vi "nanocal -- nuclear schottky fit V4.vi"() -> ()   [LabVIEW 2020] (continued)
\"B\"-> 12.000000000000  , \"θ\"-> 30.000000000000  |>   , \r\"IDS0302_210831_RAW_cal__sam_\" ->   <| \"ζ\"->  0.072634365939  , \"τ1\"-> 0.028637109000  , \"τS\"-> 0.065061142288  , \"τN\"-> 0.040304243071  , \"τC\"-> 0.001622979999  , \"κ0\"-> 0.000000001498  , \"mm1\"-> 0.000000000000  , \"mm2\"-> 0.000000000000  , \"mm3\"-> 0.000000000000  , \"T\"->  0.250000000000  , \"B\"-> 12.000000000000  , \"θ\"-> 30.000000000000  |>   , \r\"IDS0303_210831_RAW_cal__ref_\" ->   <| \"ζ\"->  0.210185455037  , \"τ1\"-> 0.035884437188  , \"τS\"-> 0.076269858590  , \"τN\"-> 0.100000000000  , \"τC\"-> 0.001092094788  , \"κ0\"-> 0.000000001049  , \"mm1\"-> 0.000000000000  , \"mm2\"-> 0.000000000000  , \"mm3\"-> 0.000000000000  , \"T\"->  0.200000000000  , \"B\"-> 12.000000000000  , \"θ\"-> 30.000000000000  |>   , \r\"IDS0303_210831_RAW_cal__sam_\" ->   <| \"ζ\"->  0.128615765969  , \"τ1\"-> 0.032665502211  , \"τS\"-> 0.082694869013  , \"τN\"-> 0.105788373632  , \"τC\"-> 0.001439686784  , \"κ0\"-> 0.000000001168  , \"mm1\"-> 0.000000000000  , \"mm2\"-> 0.000000000000  , \"mm3\"-> 0.000000000000  , \"T\"->  0.200000000000  , \"B\"-> 12.000000000000  , \"θ\"-> 30.000000000000  |>   , \r\"IDS0304_210831_RAW_cal__ref_\" ->   <| \"ζ\"->  0.270205686716  , \"τ1\"-> 0.041964859676  , \"τS\"-> 0.093295997771  , \"τN\"-> 0.171907220186  , \"τC\"-> 0.001079705974  , \"κ0\"-> 0.000000000759  , \"mm1\"-> 0.000000000000  , \"mm2\"-> 0.000000000000  , \"mm3\"-> 0.000000000000  , \"T\"->  0.170000000000  , \"B\"-> 12.000000000000  , \"θ\"-> 30.000000000000  |>   , \r\"IDS0304_210831_RAW_cal__sam_\" ->   <| \"ζ\"->  0.156472219566  , \"τ1\"-> 0.031017925061  , \"τS\"-> 0.080872234530  , \"τN\"-> 0.219381306397  , \"τC\"-> 0.001437792153  , \"κ0\"-> 0.000000000867  , \"mm1\"-> 0.000000000000  , \"mm2\"-> 0.000000000000  , \"mm3\"-> 0.000000000000  , \"T\"->  0.170000000000  , \"B\"-> 12.000000000000  , \"θ\"-> 30.000000000000  |>   , \r\"IDS0305_210831_RAW_cal__ref_\" ->   <| \"ζ\"->  0.288872243536  , \"τ1\"-> 0.043051365220  , \"τS\"-> 0.113757726379  , \"τN\"-> 0.232280670982  , \"τC\"-> 0.001075362358  , \"κ0\"-> 0.000000000648  , \"mm1\"-> 0.000000000000  , \"mm2\"-> 0.000000000000  , \"mm3\"-> 0.000000000000  , \"T\"->  0.160000000000  , \"B\"-> 12.000000000000  , \"θ\"-> 30.000000000000  |>   , \r\"IDS0305_210831_RAW_cal__sam_\" ->   <| \"ζ\"->  0.162585495535  , \"τ1\"-> 0.037883389730  , \"τS\"-> 0.086562863191  , \"τN\"-> 0.241872534356  , \"τC\"-> 0.001506143871  , \"κ0\"-> 0.000000000791  , \"mm1\"-> 0.000000000000  , \"mm2\"-> 0.000000000000  , \"mm3\"-> 0.000000000000  , \"T\"->  0.160000000000  , \"B\"-> 12.000000000000  , \"θ\"-> 30.000000000000  |>   , \r\"IDS0306_210831_RAW_cal__ref_\" ->   <| \"ζ\"->  0.013593052641  , \"τ1\"-> 0.010989385662  , \"τS\"-> 0.007947176041  , \"τN\"-> 0.000037757079  , \"τC\"-> 0.003572854733  , \"κ0\"-> 0.000000023548  , \"mm1\"-> 0.000000000000  , \"mm2\"-> 0.000000000000  , \"mm3\"-> 0.000000000000  , \"T\"->  3.100000000000  , \"B\"-> 12.000000000000  , \"θ\"-> 30.000000000000  |>   , \r\"IDS0306_210831_RAW_cal__sam_\" ->   <| \"ζ\"->  0.010111127240  , \"τ1\"-> 0.020788755574  , \"τS\"-> 0.009968978424  , \"τN\"-> 0.000077788811  , \"τC\"-> 0.004598584548  , \"κ0\"-> 0.000000024346  , \"mm1\"-> 0.000000000000  , \"mm2\"-> 0.000000000000  , \"mm3\"-> 0.000000000000  , \"T\"->  3.100000000000  , \"B\"-> 12.000000000000  , \"θ\"-> 30.000000000000  |>   , \r\"IDS0310_210901_RAW_cal__ref_\" ->   <| \"ζ\"->  0.308289315544  , \"τ1\"-> 0.054346075620  , \"τS\"-> 0.066318547481  , \"τN\"-> 0.209207967486  , \"τC\"-> 0.001005266633  , \"κ0\"-> 0.000000000648  , \"mm1\"-> 0.000000000000  , \"mm2\"-> 0.000000000000  , \"mm3\"-> 0.000000000000  , \"T\"->  0.157000000000  , \"B\"-> 12.000000000000  , \"θ\"-> 45.000000000000  |>   , \r\"IDS0310_210901_RAW_cal__sam_\" ->   <| \"ζ\"->  0.295520923520  , \"τ1\"-> 0.054772440405  , \"τS\"-> 0.071814005451  , \"τN\"-> 0.249593767169  , \"τC\"-> 0.001103632155  , \"κ0\"-> 0.000000000625  , \"mm1\"-> 0.000000000000  , \"mm2\"-> 0.000000000000  , \"mm3\"-> 0.000000000000  , \"T\"->  0.157000000000  , \"B\"-> 12.000000000000  , \"θ\"-> 45.000000000000  |>   , \r\"IDS0311_210901_RAW_cal__ref_\" ->   <| \"ζ\"->  0.509291398058  , \"τ1\"-> 0.072489311123  , \"τS\"-> 0.090971238975  , \"τN\"-> 0.493344947632  , \"τC\"-> 0.000983845591  , \"κ0\"-> 0.000000000427  , \"mm1\"-> 0.000000000000  , \"mm2\"-> 0.000000000000  , \"mm3\"-> 0.000000000000  , \"T\"->  0.120000000000  , \"B\"-> 12.000000000000  , \"θ\"-> 45.000000000000  |>   , \r\"IDS0311_210901_RAW_cal__sam_\" ->   <| \"ζ\"->  0.523545279740  , \"τ1\"-> 0.065613539167  , \"τS\"-> 0.100000000000  , \"τN\"-> 0.424083114177  , \"τC\"-> 0.000911255863  , \"κ0\"-> 0.000000000418  , \"mm1\"-> 0.000000000000  , \"mm2\"-> 0.000000000000  , \"mm3\"-> 0.000000000000  , \"T\"->  0.120000000000  , \"B\"-> 12.000000000000  , \"θ\"-> 45.000000000000  |>   , \r\"IDS0312_210901_RAW_cal__ref_\" ->   <| \"ζ\"->  0.255987747016  , \"τ1\"-> 0.050915418179  , \"τS\"-> 0.056322890077  , \"τN\"-> 0.162539494258  , \"τC\"-> 0.001014478551  , \"κ0\"-> 0.000000000752  , \"mm1\"-> 0.000000000000  , \"mm2\"-> 0.000000000000  , \"mm3\"-> 0.000000000000  , \"T\"->  0.170000000000  , \"B\"-> 12.000000000000  , \"θ\"-> 45.000000000000  |>   , \r\"IDS0312_210901_RAW_cal__sam_\" ->   <| \"ζ\"->  0.273742116471  , \"τ1\"-> 0.052262909995  , \"τS\"-> 0.060554036646  , \"τN\"-> 0.154269705680  , \"τC\"-> 0.001074144337  , \"κ0\"-> 0.000000000753  , \"mm1\"-> 0.000000000000  , \"mm2\"-> 0.000000000000  , \"mm3\"-> 0.000000000000  , \"T\"->  0.170000000000  , \"B\"-> 12.000000000000  , \"θ\"-> 45.000000000000  |>   , \r\"IDS0313_210901_RAW_cal__ref_\" ->   <| \"ζ\"->  0.214174227031  , \"τ1\"-> 0.045371966885  , \"τS\"-> 0.046160741010  , \"τN\"-> 0.090352099204  , \"τC\"-> 0.001077653985  , \"κ0\"-> 0.000000001047  , \"mm1\"-> 0.000000000000  , \"mm2\"-> 0.000000000000  , \"mm3\"-> 0.000000000000  , \"T\"->  0.200000000000  , \"B\"-> 12.000000000000  , \"θ\"-> 45.000000000000  |>   , \r\"IDS0313_210901_RAW_cal__sam_\" ->   <| \"ζ\"->  0.215688135788  , \"τ1\"-> 0.043710888546  , \"τS\"-> 0.044756474141  , \"τN\"-> 0.090222547904  , \"τC\"-> 0.001049781785  , \"κ0\"-> 0.000000001047  , \"mm1\"-> 0.000000000000  , \"mm2\"-> 0.000000000000  , \"mm3\"-> 0.000000000000  , \"T\"->  0.200000000000  , \"B\"-> 12.000000000000  , \"θ\"-> 45.000000000000  |>   , \r\"IDS0314_210901_RAW_cal__ref_\" ->   <| \"ζ\"->  0.121938807235  , \"τ1\"-> 0.034207371807  , \"τS\"-> 0.036720955072  , \"τN\"-> 0.033836278502  , \"τC\"-> 0.001295467245  , \"κ0\"-> 0.000000001354  , \"mm1\"-> 0.000000000000  , \"mm2\"-> 0.000000000000  , \"mm3\"-> 0.000000000000  , \"T\"->  0.255000000000  , \"B\"-> 12.000000000000  , \"θ\"-> 45.000000000000  |>   , \r\"IDS0314_210901_RAW_cal__sam_\" ->   <| \"ζ\"->  0.118583992968  , \"τ1\"-> 0.035232851003  , \"τS\"-> 0.037458022816  , \"τN\"-> 0.033724509363  , \"τC\"-> 0.001440922263  , \"κ0\"-> 0.000000001360  , \"mm1\"-> 0.000000000000  , \"mm2\"-> 0.000000000000  , \"mm3\"-> 0.000000000000  , \"T\"->  0.255000000000  , \"B\"-> 12.000000000000  , \"θ\"-> 45.000000000000  |>   , \r\"IDS0315_210901_RAW_cal__ref_\" ->   <| \"ζ\"->  0.083994348522  , \"τ1\"-> 0.028454655874  , \"τS\"-> 0.032547522861  , \"τN\"-> 0.016695645368  , \"τC\"-> 0.001519868181  , \"κ0\"-> 0.000000001732  , \"mm1\"-> 0.000000000000  , \"mm2\"-> 0.000000000000  , \"mm3\"-> 0.000000000000  , \"T\"->  0.300000000000  , \"B\"-> 12.000000000000  , \"θ\"-> 45.000000000000  |>   , \r\"IDS0315_210901_RAW_cal__sam_\" ->   <| \"ζ\"->  0.085152769414  , \"τ1\"-> 0.029001116263  , \"τS\"-> 0.032604663993  , \"τN\"-> 0.016878763935  , \"τC\"-> 0.001443524845  , \"κ0\"-> 0.000000001728  , \"mm1\"-> 0.000000000000  , \"mm2\"-> 0.000000000000  , \"mm3\"-> 0.000000000000  , \"T\"->  0.300000000000  , \"B\"-> 12.000000000000  , \"θ\"-> 45.000000000000  |>   , \r\"IDS0316_210901_RAW_cal__ref_\" ->   <| \"ζ\"->  0.061161812807  , \"τ1\"-> 0.025679940958  , \"τS\"-> 0.030186846656  , \"τN\"-> 0.009745770789  , \"τC\"-> 0.001942458613  , \"κ0\"-> 0.000000002119  , \"mm1\"-> 0.000000000000  , \"mm2\"-> 0.000000000000  , \"mm3\"-> 0.000000000000  , \"T\"->  0.360000000000  , \"B\"-> 12.000000000000  , \"θ\"-> 45.000000000000  |>   , \r\"IDS0316_210901_RAW_cal__sam_\" ->   <| \"ζ\"->  0.061011838044  , \"τ1\"-> 0.025440548989  , \"τS\"-> 0.030028053978  , \"τN\"-> 0.010140731955  , \"τC\"-> 0.001895079687  , \"κ0\"-> 0.000000002115  , \"mm1\"-> 0.000000000000  , \"mm2\"-> 0.000000000000  , \"mm3\"-> 0.000000000000  , \"T\"->  0.360000000000  , \"B\"-> 12.000000000000  , \"θ\"-> 45.000000000000  |>   , \r\"IDS0317_210901_RAW_cal__ref_\" ->   <| \"ζ\"->  0.047188818117  , \"τ1\"-> 0.023281630947  , \"τS\"-> 0.027595934693  , \"τN\"-> 0.005357909158  , \"τC\"-> 0.002405018291  , \"κ0\"-> 0.000000002634  , \"mm1\"-> 0.000000000000  , \"mm2\"-> 0.000000000000  , \"mm3\"-> 0.000000000000  , \"T\"->  0.430000000000  , \"B\"-> 12.000000000000  , \"θ\"-> 45.000000000000  |>   , \r\"IDS0317_210901_RAW_cal__sam_\" ->   <| \"ζ\"->  0.046686299518  , \"τ1\"-> 0.021011215626  , \"τS\"-> 0.027633142317  , \"τN\"-> 0.005348477555  , \"τC\"-> 0.002098477650  , \"κ0\"-> 0.000000002635  , \"mm1\"-> 0.000000000000  , \"mm2\"-> 0.000000000000  , \"mm3\"-> 0.000000000000  , \"T\"->  0.430000000000  , \"B\"-> 12.000000000000  , \"θ\"-> 45.000000000000  |>   , \r\"IDS0318_210901_RAW_cal__ref_\" ->   <| \"ζ\"->  0.037288247068  , \"τ1\"-> 0.020701608824  , \"τS\"-> 0.025512873362  , \"τN\"-> 0.002622201076  , \"τC\"-> 0.002753838304  , \"κ0\"-> 0.000000003290  , \"mm1\"-> 0.000000000000  , \"mm2\"-> 0.000000000000  , \"mm3\"-> 0.000000000000  , \"T\"->  0.530000000000  , \"B\"-> 12.000000000000  , \"θ\"-> 45.000000000000  |>   , \r\"IDS0318_210901_RAW_cal__sam_\" ->   <| \"ζ\"->  0.035204330012  , \"τ1\"-> 0.021011523093  , \"τS\"-> 0.025247316079  , \"τN\"-> 0.002718647875  , \"τC\"-> 0.003091727575  , \"κ0\"-> 0.000000003296  , \"mm1\"-> 0.000000000000  , \"mm2\"-> 0.000000000000  , \"mm3\"-> 0.000000000000  , \"T\"->  0.530000000000  , \"B\"-> 12.000000000000  , \"θ\"-> 45.000000000000  |>   , \r\"IDS0319_210901_RAW_cal__ref_\" ->   <| \"ζ\"->  0.029057248634  , \"τ1\"-> 0.018506971535  , \"τS\"-> 0.023958337181  , \"τN\"-> 0.001609750825  , \"τC\"-> 0.003041346082  , \"κ0\"-> 0.000000003909  , \"mm1\"-> 0.000000000000  , \"mm2\"-> 0.000000000000  , \"mm3\"-> 0.000000000000  , \"T\"->  0.620000000000  , \"B\"-> 12.000000000000  , \"θ\"-> 45.000000000000  |>   , \r\"IDS0319_210901_RAW_cal__sam_\" ->   <| \"ζ\"->  0.030862035723  , \"τ1\"-> 0.019328530751  , \"τS\"-> 0.023568572597  , \"τN\"-> 0.001701966614  , \"τC\"-> 0.003453790534  , \"κ0\"-> 0.000000003906  , \"mm1\"-> 0.000000000000  , \"mm2\"-> 0.000000000000  , \"mm3\"-> 0.000000000000  , \"T\"->  0.620000000000  , \"B\"-> 12.000000000000  , \"θ\"-> 45.000000000000  |>   , \r\"IDS0320_210901_RAW_cal__ref_\" ->   <| \"ζ\"->  0.022379315068  , \"τ1\"-> 0.015662672554  , \"τS\"-> 0.020062485201  , \"τN\"-> 0.000750608517  , \"τC\"-> 0.004162319228  , \"κ0\"-> 0.000000005449  , \"mm1\"-> 0.000000000000  , \"mm2\"-> 0.000000000000  , \"mm3\"-> 0.000000000000  , \"T\"->  0.830000000000  , \"B\"-> 12.000000000000  , \"θ\"-> 45.000000000000  |>   , \r\"IDS0320_210901_RAW_cal__sam_\" ->   <| \"ζ\"->  0.023591124045  , \"τ1\"-> 0.014910006225  , \"τS\"-> 0.019342950404  , \"τN\"-> 0.000752972387  , \"τC\"-> 0.004900413232  , \"κ0\"-> 0.000000005453  , \"mm1\"-> 0.000000000000  , \"mm2\"-> 0.000000000000  , \"mm3\"-> 0.000000000000  , \"T\"->  0.830000000000  , \"B\"-> 12.000000000000  , \"θ\"-> 45.000000000000  |>   , \r\"IDS0321_210901_RAW_cal__ref_\" ->   <| \"ζ\"->  0.020614746765  , \"τ1\"-> 0.013682065369  , \"τS\"-> 0.016105139108  , \"τN\"-> 0.000397734649  , \"τC\"-> 0.005005824303  , \"κ0\"-> 0.000000007592  , \"mm1\"-> 0.000000000000  , \"mm2\"-> 0.000000000000  , \"mm3\"-> 0.000000000000  , \"T\"->  1.130000000000  , \"B\"-> 12.000000000000  , \"θ\"-> 45.000000000000  |>   , \r\"IDS0321_210901_RAW_cal__sam_\" ->   <| \"ζ\"->  0.020215154826  , \"τ1\"-> 0.014105227254  , \"τS\"-> 0.015660924043  , \"τN\"-> 0.000525137036  , \"τC\"-> 0.005447728357  , \"κ0\"-> 0.000000007594  , \"mm1\"-> 0.000000000000  , \"mm2\"-> 0.000000000000  , \"mm3\"-> 0.000000000000  , \"T\"->  1.130000000000  , \"B\"-> 12.000000000000  , \"θ\"-> 45.000000000000  |>   , \r\"IDS0322_210901_RAW_cal__ref_\" ->   <| \"ζ\"->  0.019557893298  , \"τ1\"-> 0.012446212333  , \"τS\"-> 0.011139553358  , \"τN\"-> 0.000114229396  , \"τC\"-> 0.005115315079  , \"κ0\"-> 0.000000013115  , \"mm1\"-> 0.000000000000  , \"mm2\"-> 0.000000000000  , \"mm3\"-> 0.000000000000  , \"T\"->  1.900000000000  , \"B\"-> 12.000000000000  , \"θ\"-> 45.000000000000  |>   , \r\"IDS0322_210901_RAW_cal__sam_\" ->   <| \"ζ\"->  0.018090572724  , \"τ1\"-> 0.013314780956  , \"τS\"-> 0.010820835010  , \"τN\"-> 0.000265552167  , \"τC\"-> 0.005393540417  , \"κ0\"-> 0.000000013100  , \"mm1\"-> 0.000000000000  , \"mm2\"-> 0.000000000000  , \"mm3\"-> 0.000000000000  , \"T\"->  1.900000000000  , \"B\"-> 12.000000000000  , \"θ\"-> 45.000000000000  |>   , \r\"IDS0323_210901_RAW_cal__ref_\" ->   <| \"ζ\"->  0.018290634783  , \"τ1\"-> 0.011707989393  , \"τS\"-> 0.007391181448  , \"τN\"-> 0.000042685582  , \"τC\"-> 0.004638632451  , \"κ0\"-> 0.000000023525  , \"mm1\"-> 0.000000000000  , \"mm2\"-> 0.000000000000  , \"mm3\"-> 0.000000000000  , \"T\"->  3.100000000000  , \"B\"-> 12.000000000000  , \"θ\"-> 45.000000000000  |>   , \r\"IDS0323_210901_RAW_cal__sam_\" ->   <| \"ζ\"->  0.019438138135  , \"τ1\"-> 0.013521019406  , \"τS\"-> 0.007253169401  , \"τN\"-> 0.000154824830  , \"τC\"-> 0.004746579385  , \"κ0\"-> 0.000000023466  , \"mm1\"-> 0.000000000000  , \"mm2\"-> 0.000000000000  , \"mm3\"-> 0.000000000000  , \"T\"->  3.100000000000  , \"B\"-> 12.000000000000  , \"θ\"-> 45.000000000000  |>   , \r\"IDS0324_210901_RAW_cal__ref_\" ->   <| \"ζ\"->  0.016342153608  , \"τ1\"-> 0.012470308436  , \"τS\"-> 0.004793459347  , \"τN\"-> 0.000012881713  , \"τC\"-> 0.003213848745  , \"κ0\"-> 0.000000058321  , \"mm1\"-> 0.000000000000  , \"mm2\"-> 0.000000000000  , \"mm3\"-> 0.000000000000  , \"T\"->  5.700000000000  , \"B\"-> 12.000000000000  , \"θ\"-> 45.000000000000  |>   , \r\"IDS0324_210901_RAW_cal__sam_\" ->   <| \"ζ\"->  0.018573189054  , \"τ1\"-> 0.013304612245  , \"τS\"-> 0.003723860844  , \"τN\"-> 0.000084829442  , \"τC\"-> 0.004309703632  , \"κ0\"-> 0.000000058362  , \"mm1\"-> 0.000000000000  , \"mm2\"-> 0.000000000000  , \"mm3\"-> 0.000000000000  , \"T\"->  5.700000000000  , \"B\"-> 12.000000000000  , \"θ\"-> 45.000000000000  |>   , \r\"IDS0330_210901_RAW_cal__ref_\" ->   <| \"ζ\"->  0.000000000000  , \"τ1\"-> 0.000000000000  , \"τS\"-> 0.000000000000  , \"τN\"-> 0.000000000000  , \"τC\"-> 0.000000000000  , \"κ0\"-> 0.000000000000  , \"mm1\"-> 0.000000000000  , \"mm2\"-> 0.000000000000  , \"mm3\"-> 0.000000000000  , \"T\"->  0.197000000000  , \"B\"-> 1.000000000000  , \"θ\"-> 90.000000000000  |>   , \r\"IDS0330_210901_RAW_cal__sam_\" ->   <| \"ζ\"->  0.000000000000  , \"τ1\"-> 0.000000000000  , \"τS\"-> 0.000000000000  , \"τN\"-> 0.000000000000  , \"τC\"-> 0.000000000000  , \"κ0\"-> 0.000000000000  , \"mm1\"-> 0.000000000000  , \"mm2\"-> 0.000000000000  , \"mm3\"-> 0.000000000000  , \"T\"->  0.197000000000  , \"B\"-> 1.000000000000  , \"θ\"-> 90.000000000000  |>   , \r\"IDS0331_210901_RAW_cal__ref_\" ->   <| \"ζ\"->  0.000000000000  , \"τ1\"-> 0.000000000000  , \"τS\"-> 0.000000000000  , \"τN\"-> 0.000000000000  , \"τC\"-> 0.000000000000  , \"κ0\"-> 0.000000000000  , \"mm1\"-> 0.000000000000  , \"mm2\"-> 0.000000000000  , \"mm3\"-> 0.000000000000  , \"T\"->  0.197000000000  , \"B\"-> 2.000000000000  , \"θ\"-> 90.000000000000  |>   , \r\"IDS0331_210901_RAW_cal__sam_\" ->   <| \"ζ\"->  0.000000000000  , \"τ1\"-> 0.000000000000  , \"τS\"-> 0.000000000000  , \"τN\"-> 0.000000000000  , \"τC\"-> 0.000000000000  , \"κ0\"-> 0.000000000000  , \"mm1\"-> 0.000000000000  , \"mm2\"-> 0.000000000000  , \"mm3\"-> 0.000000000000  , \"T\"->  0.197000000000  , \"B\"-> 2.000000000000  , \"θ\"-> 90.000000000000  |>   , \r\"IDS0335_210904_RAW_cal__ref_\" ->   <| \"ζ\"->  0.205498470214  , \"τ1\"-> 0.028285232133  , \"τS\"-> 0.084091632013  , \"τN\"-> 0.011152237921  , \"τC\"-> 0.001130624685  , \"κ0\"-> 0.000000001029  , \"mm1\"-> 0.000000000000  , \"mm2\"-> 0.000000000000  , \"mm3\"-> 0.000000000000  , \"T\"->  0.197000000000  , \"B\"-> 5.000000000000  , \"θ\"-> 90.000000000000  |>   , \r\"IDS0335_210904_RAW_cal__sam_\" ->   <| \"ζ\"->  0.126020527573  , \"τ1\"-> 0.019611338518  , \"τS\"-> 0.107746773503  , \"τN\"-> 0.016174642295  , \"τC\"-> 0.001503883282  , \"κ0\"-> 0.000000001131  , \"mm1\"-> 0.000000000000  , \"mm2\"-> 0.000000000000  , \"mm3\"-> 0.000000000000  , \"T\"->  0.197000000000  , \"B\"-> 5.000000000000  , \"θ\"-> 90.000000000000  |>   , \r\"IDS0336_210904_RAW_cal__ref_\" ->   <| \"ζ\"->  0.375717568518  , \"τ1\"-> 0.027671879302  , \"τS\"-> 0.199029510980  , \"τN\"-> 0.083427621052  , \"τC\"-> 0.001244823236  , \"κ0\"-> 0.000000000403  , \"mm1\"-> 0.000000000000  , \"mm2\"-> 0.000000000000  , \"mm3\"-> 0.000000000000  , \"T\"->  0.122000000000  , \"B\"-> 5.000000000000  , \"θ\"-> 90.000000000000  |>   , \r\"IDS0336_210904_RAW_cal__sam_\" ->   <| \"ζ\"->  0.199029510980  , \"τ1\"-> 0.022641147583  , \"τS\"-> 0.278068103221  , \"τN\"-> 0.092231648139  , \"τC\"-> 0.001612694918  , \"κ0\"-> 0.000000000500  , \"mm1\"-> 0.000000000000  , \"mm2\"-> 0.000000000000  , \"mm3\"-> 0.000000000000  , \"T\"->  0.122000000000  , \"B\"-> 5.000000000000  , \"θ\"-> 90.000000000000  |>   , \r\"IDS0337_210904_RAW_cal__ref_\" ->   <| \"ζ\"->  0.292356831523  , \"τ1\"-> 0.026984636460  , \"τS\"-> 0.124002379909  , \"τN\"-> 0.023667494338  , \"τC\"-> 0.001131071001  , \"κ0\"-> 0.000000000646  , \"mm1\"-> 0.000000000000  , \"mm2\"-> 0.000000000000  , \"mm3\"-> 0.000000000000  , \"T\"->  0.157000000000  , \"B\"-> 5.000000000000  , \"θ\"-> 90.000000000000  |>   , \r\"IDS0337_210904_RAW_cal__sam_\" ->   <| \"ζ\"->  0.176509782472  , \"τ1\"-> 0.020702853275  , \"τS\"-> 0.157609352978  , \"τN\"-> 0.029245874633  , \"τC\"-> 0.001454463496  , \"κ0\"-> 0.000000000745  , \"mm1\"-> 0.000000000000  , \"mm2\"-> 0.000000000000  , \"mm3\"-> 0.000000000000  , \"T\"->  0.157000000000  , \"B\"-> 5.000000000000  , \"θ\"-> 90.000000000000  |>   , \r\"IDS0338_210904_RAW_cal__ref_\" ->   <| \"ζ\"->  0.269210160049  , \"τ1\"-> 0.027533256233  , \"τS\"-> 0.109874895668  , \"τN\"-> 0.015552411517  , \"τC\"-> 0.001074349295  , \"κ0\"-> 0.000000000732  , \"mm1\"-> 0.000000000000  , \"mm2\"-> 0.000000000000  , \"mm3\"-> 0.000000000000  , \"T\"->  0.170000000000  , \"B\"-> 5.000000000000  , \"θ\"-> 90.000000000000  |>   , \r\"IDS0338_210904_RAW_cal__sam_\" ->   <| \"ζ\"->  0.165922290438  , \"τ1\"-> 0.020050534769  , \"τS\"-> 0.138657975356  , \"τN\"-> 0.024093470374  , \"τC\"-> 0.001416071995  , \"κ0\"-> 0.000000000842  , \"mm1\"-> 0.000000000000  , \"mm2\"-> 0.000000000000  , \"mm3\"-> 0.000000000000  , \"T\"->  0.170000000000  , \"B\"-> 5.000000000000  , \"θ\"-> 90.000000000000  |>   , \r\"IDS0339_210904_RAW_cal__ref_\" ->   <| \"ζ\"->  0.119201785186  , \"τ1\"-> 0.025848962424  , \"τS\"-> 0.059947037778  , \"τN\"-> 0.005199563600  , \"τC\"-> 0.001300898921  , \"κ0\"-> 0.000000001342  , \"mm1\"-> 0.000000000000  , \"mm2\"-> 0.000000000000  , \"mm3\"-> 0.000000000000  , \"T\"->  0.255000000000  , \"B\"-> 5.000000000000  , \"θ\"-> 90.000000000000  |>   , \r\"IDS0339_210904_RAW_cal__sam_\" ->   <| \"ζ\"->  0.071445093965  , \"τ1\"-> 0.018200134719  , \"τS\"-> 0.077244369618  , \"τN\"-> 0.007618519700  , \"τC\"-> 0.001758409609  , \"κ0\"-> 0.000000001475  , \"mm1\"-> 0.000000000000  , \"mm2\"-> 0.000000000000  , \"mm3\"-> 0.000000000000  , \"T\"->  0.255000000000  , \"B\"-> 5.000000000000  , \"θ\"-> 90.000000000000  |>   , \r\"IDS0340_210904_RAW_cal__ref_\" ->   <| \"ζ\"->  0.082683893253  , \"τ1\"-> 0.024702194699  , \"τS\"-> 0.049753720072  , \"τN\"-> 0.002517387539  , \"τC\"-> 0.001542602546  , \"κ0\"-> 0.000000001719  , \"mm1\"-> 0.000000000000  , \"mm2\"-> 0.000000000000  , \"mm3\"-> 0.000000000000  , \"T\"->  0.308000000000  , \"B\"-> 5.000000000000  , \"θ\"-> 90.000000000000  |>   , \r\"IDS0340_210904_RAW_cal__sam_\" ->   <| \"ζ\"->  0.049152938826  , \"τ1\"-> 0.019216107215  , \"τS\"-> 0.064101941953  , \"τN\"-> 0.003869712687  , \"τC\"-> 0.002203680801  , \"κ0\"-> 0.000000001878  , \"mm1\"-> 0.000000000000  , \"mm2\"-> 0.000000000000  , \"mm3\"-> 0.000000000000  , \"T\"->  0.308000000000  , \"B\"-> 5.000000000000  , \"θ\"-> 90.000000000000  |>   , \r\"IDS0341_210904_RAW_cal__ref_\" ->   <| \"ζ\"->  0.059616809183  , \"τ1\"-> 0.023939570797  , \"τS\"-> 0.042653632086  , \"τN\"-> 0.001786288241  , \"τC\"-> 0.001975926031  , \"κ0\"-> 0.000000002092  , \"mm1\"-> 0.000000000000  , \"mm2\"-> 0.000000000000  , \"mm3\"-> 0.000000000000  , \"T\"->  0.360000000000  , \"B\"-> 5.000000000000  , \"θ\"-> 90.000000000000  |>   , \r\"IDS0341_210904_RAW_cal__sam_\" ->   <| \"ζ\"->  0.036041476168  , \"τ1\"-> 0.019203470752  , \"τS\"-> 0.054931014880  , \"τN\"-> 0.002271152158  , \"τC\"-> 0.002720100083  , \"κ0\"-> 0.000000002280  , \"mm1\"-> 0.000000000000  , \"mm2\"-> 0.000000000000  , \"mm3\"-> 0.000000000000  , \"T\"->  0.360000000000  , \"B\"-> 5.000000000000  , \"θ\"-> 90.000000000000  |>   , \r\"IDS0342_210904_RAW_cal__ref_\" ->   <| \"ζ\"->  0.044217232361  , \"τ1\"-> 0.023574215500  , \"τS\"-> 0.035981580515  , \"τN\"-> 0.001074333911  , \"τC\"-> 0.002351862552  , \"κ0\"-> 0.000000002629  , \"mm1\"-> 0.000000000000  , \"mm2\"-> 0.000000000000  , \"mm3\"-> 0.000000000000  , \"T\"->  0.438000000000  , \"B\"-> 5.000000000000  , \"θ\"-> 90.000000000000  |>   , \r\"IDS0342_210904_RAW_cal__sam_\" ->   <| \"ζ\"->  0.027360242550  , \"τ1\"-> 0.019369895135  , \"τS\"-> 0.046063450687  , \"τN\"-> 0.001549427641  , \"τC\"-> 0.003313507267  , \"κ0\"-> 0.000000002850  , \"mm1\"-> 0.000000000000  , \"mm2\"-> 0.000000000000  , \"mm3\"-> 0.000000000000  , \"T\"->  0.438000000000  , \"B\"-> 5.000000000000  , \"θ\"-> 90.000000000000  |>   , \r\"IDS0343_210904_RAW_cal__ref_\" ->   <| \"ζ\"->  0.035616644679  , \"τ1\"-> 0.021293989016  , \"τS\"-> 0.030504656314  , \"τN\"-> 0.000733387796  , \"τC\"-> 0.002756004742  , \"κ0\"-> 0.000000003268  , \"mm1\"-> 0.000000000000  , \"mm2\"-> 0.000000000000  , \"mm3\"-> 0.000000000000  , \"T\"->  0.530000000000  , \"B\"-> 5.000000000000  , \"θ\"-> 90.000000000000  |>   , \r\"IDS0343_210904_RAW_cal__sam_\" ->   <| \"ζ\"->  0.022691746072  , \"τ1\"-> 0.019361166937  , \"τS\"-> 0.038571137960  , \"τN\"-> 0.001037489181  , \"τC\"-> 0.004002961022  , \"κ0\"-> 0.000000003536  , \"mm1\"-> 0.000000000000  , \"mm2\"-> 0.000000000000  , \"mm3\"-> 0.000000000000  , \"T\"->  0.530000000000  , \"B\"-> 5.000000000000  , \"θ\"-> 90.000000000000  |>   , \r\"IDS0344_210904_RAW_cal__ref_\" ->   <| \"ζ\"->  0.029414072191  , \"τ1\"-> 0.022729389588  , \"τS\"-> 0.026807996891  , \"τN\"-> 0.000501873075  , \"τC\"-> 0.003020821681  , \"κ0\"-> 0.000000003880  , \"mm1\"-> 0.000000000000  , \"mm2\"-> 0.000000000000  , \"mm3\"-> 0.000000000000  , \"T\"->  0.620000000000  , \"B\"-> 5.000000000000  , \"θ\"-> 90.000000000000  |>   , \r\"IDS0344_210904_RAW_cal__sam_\" ->   <| \"ζ\"->  0.018598309928  , \"τ1\"-> 0.019376212159  , \"τS\"-> 0.033569863125  , \"τN\"-> 0.000771760425  , \"τC\"-> 0.004371934540  , \"κ0\"-> 0.000000004218  , \"mm1\"-> 0.000000000000  , \"mm2\"-> 0.000000000000  , \"mm3\"-> 0.000000000000  , \"T\"->  0.620000000000  , \"B\"-> 5.000000000000  , \"θ\"-> 90.000000000000  |>   , \r\"IDS0346_210904_RAW_cal__ref_\" ->   <| \"ζ\"->  0.351410523880  , \"τ1\"-> 0.038660935015  , \"τS\"-> 0.057750106762  , \"τN\"-> 0.192483765517  , \"τC\"-> 0.000883347451  , \"κ0\"-> 0.000000000403  , \"mm1\"-> 0.000000000000  , \"mm2\"-> 0.000000000000  , \"mm3\"-> 0.000000000000  , \"T\"->  0.122000000000  , \"B\"-> 8.000000000000  , \"θ\"-> 90.000000000000  |>   , \r\"IDS0346_210904_RAW_cal__sam_\" ->   <| \"ζ\"->  0.000000000000  , \"τ1\"-> 0.000000000000  , \"τS\"-> 0.000000000000  , \"τN\"-> 0.000000000000  , \"τC\"-> 0.000000000000  , \"κ0\"-> 0.000000000000  , \"mm1\"-> 0.000000000000  , \"mm2\"-> 0.000000000000  , \"mm3\"-> 0.000000000000  , \"T\"->  0.122000000000  , \"B\"-> 8.000000000000  , \"θ\"-> 90.000000000000  |>   , \r\"IDS0347_210906_RAW_cal__ref_\" ->   <| \"ζ\"->  0.282365663511  , \"τ1\"-> 0.039144945999  , \"τS\"-> 0.059953399264  , \"τN\"-> 0.108048405778  , \"τC\"-> 0.001096068963  , \"κ0\"-> 0.000000000641  , \"mm1\"-> 0.000000000000  , \"mm2\"-> 0.000000000000  , \"mm3\"-> 0.000000000000  , \"T\"->  0.157000000000  , \"B\"-> 8.000000000000  , \"θ\"-> 90.000000000000  |>   , \r\"IDS0347_210906_RAW_cal__sam_\" ->   <| \"ζ\"->  0.000000000000  , \"τ1\"-> 0.000000000000  , \"τS\"-> 0.000000000000  , \"τN\"-> 0.000000000000  , \"τC\"-> 0.000000000000  , \"κ0\"-> 0.000000000000  , \"mm1\"-> 0.000000000000  , \"mm2\"-> 0.000000000000  , \"mm3\"-> 0.000000000000  , \"T\"->  0.157000000000  , \"B\"-> 8.000000000000  , \"θ\"-> 90.000000000000  |>   , \r\"IDS0348_210906_RAW_cal__ref_\" ->   <| \"ζ\"->  0.231232733983  , \"τ1\"-> 0.036430431380  , \"τS\"-> 0.054781597050  , \"τN\"-> 0.064844477869  , \"τC\"-> 0.001068830966  , \"κ0\"-> 0.000000000760  , \"mm1\"-> 0.000000000000  , \"mm2\"-> 0.000000000000  , \"mm3\"-> 0.000000000000  , \"T\"->  0.178000000000  , \"B\"-> 8.000000000000  , \"θ\"-> 90.000000000000  |>   , \r\"IDS0348_210906_RAW_cal__sam_\" ->   <| \"ζ\"->  0.000000000000  , \"τ1\"-> 0.000000000000  , \"τS\"-> 0.000000000000  , \"τN\"-> 0.000000000000  , \"τC\"-> 0.000000000000  , \"κ0\"-> 0.000000000000  , \"mm1\"-> 0.000000000000  , \"mm2\"-> 0.000000000000  , \"mm3\"-> 0.000000000000  , \"T\"->  0.178000000000  , \"B\"-> 8.000000000000  , \"θ\"-> 90.000000000000  |>   , \r\"IDS0349_210906_RAW_cal__ref_\" ->   <| \"ζ\"->  0.190485473901  , \"τ1\"-> 0.032323616024  , \"τS\"-> 0.052823523941  , \"τN\"-> 0.036537332757  , \"τC\"-> 0.001181014846  , \"κ0\"-> 0.000000001037  , \"mm1\"-> 0.000000000000  , \"mm2\"-> 0.000000000000  , \"mm3\"-> 0.000000000000  , \"T\"->  0.200000000000  , \"B\"-> 8.000000000000  , \"θ\"-> 90.000000000000  |>   , \r\"IDS0349_210906_RAW_cal__sam_\" ->   <| \"ζ\"->  0.000000000000  , \"τ1\"-> 0.000000000000  , \"τS\"-> 0.000000000000  , \"τN\"-> 0.000000000000  , \"τC\"-> 0.000000000000  , \"κ0\"-> 0.000000000000  , \"mm1\"-> 0.000000000000  , \"mm2\"-> 0.000000000000  , \"mm3\"-> 0.000000000000  , \"T\"->  0.200000000000  , \"B\"-> 8.000000000000  , \"θ\"-> 90.000000000000  |>   , \r\"IDS0350_210906_RAW_cal__ref_\" ->   <| \"ζ\"->  0.118733755426  , \"τ1\"-> 0.027090622935  , \"τS\"-> 0.042154952610  , \"τN\"-> 0.016299612233  , \"τC\"-> 0.001268322773  , \"κ0\"-> 0.000000001347  , \"mm1\"-> 0.000000000000  , \"mm2\"-> 0.000000000000  , \"mm3\"-> 0.000000000000  , \"T\"->  0.260000000000  , \"B\"-> 8.000000000000  , \"θ\"-> 90.000000000000  |>   , \r\"IDS0350_210906_RAW_cal__sam_\" ->   <| \"ζ\"->  0.000000000000  , \"τ1\"-> 0.000000000000  , \"τS\"-> 0.000000000000  , \"τN\"-> 0.000000000000  , \"τC\"-> 0.000000000000  , \"κ0\"-> 0.000000000000  , \"mm1\"-> 0.000000000000  , \"mm2\"-> 0.000000000000  , \"mm3\"-> 0.000000000000  , \"T\"->  0.260000000000  , \"B\"-> 8.000000000000  , \"θ\"-> 90.000000000000  |>   , \r\"IDS0351_210906_RAW_cal__ref_\" ->   <| \"ζ\"->  0.081031099964  , \"τ1\"-> 0.021876847581  , \"τS\"-> 0.037173038366  , \"τN\"-> 0.007845971856  , \"τC\"-> 0.001561862252  , \"κ0\"-> 0.000000001761  , \"mm1\"-> 0.000000000000  , \"mm2\"-> 0.000000000000  , \"mm3\"-> 0.000000000000  , \"T\"->  0.310000000000  , \"B\"-> 8.000000000000  , \"θ\"-> 90.000000000000  |>   , \r\"IDS0351_210906_RAW_cal__sam_\" ->   <| \"ζ\"->  0.000000000000  , \"τ1\"-> 0.000000000000  , \"τS\"-> 0.000000000000  , \"τN\"-> 0.000000000000  , \"τC\"-> 0.000000000000  , \"κ0\"-> 0.000000000000  , \"mm1\"-> 0.000000000000  , \"mm2\"-> 0.000000000000  , \"mm3\"-> 0.000000000000  , \"T\"->  0.310000000000  , \"B\"-> 8.000000000000  , \"θ\"-> 90.000000000000  |>   , \r\"IDS0352_210906_RAW_cal__ref_\" ->   <| \"ζ\"->  0.060336863550  , \"τ1\"-> 0.020607625563  , \"τS\"-> 0.034334079822  , \"τN\"-> 0.004923011954  , \"τC\"-> 0.001895452704  , \"κ0\"-> 0.000000002106  , \"mm1\"-> 0.000000000000  , \"mm2\"-> 0.000000000000  , \"mm3\"-> 0.000000000000  , \"T\"->  0.360000000000  , \"B\"-> 8.000000000000  , \"θ\"-> 90.000000000000  |>   , \r\"IDS0352_210906_RAW_cal__sam_\" ->   <| \"ζ\"->  0.000000000000  , \"τ1\"-> 0.000000000000  , \"τS\"-> 0.000000000000  , \"τN\"-> 0.000000000000  , \"τC\"-> 0.000000000000  , \"κ0\"-> 0.000000000000  , \"mm1\"-> 0.000000000000  , \"mm2\"-> 0.000000000000  , \"mm3\"-> 0.000000000000  , \"T\"->  0.360000000000  , \"B\"-> 8.000000000000  , \"θ\"-> 90.000000000000  |>   , \r\"IDS0353_210906_RAW_cal__ref_\" ->   <| \"ζ\"->  0.045012118583  , \"τ1\"-> 0.020623291685  , \"τS\"-> 0.031197986163  , \"τN\"-> 0.002724775132  , \"τC\"-> 0.002225741907  , \"κ0\"-> 0.000000002626  , \"mm1\"-> 0.000000000000  , \"mm2\"-> 0.000000000000  , \"mm3\"-> 0.000000000000  , \"T\"->  0.438000000000  , \"B\"-> 8.000000000000  , \"θ\"-> 90.000000000000  |>   , \r\"IDS0353_210906_RAW_cal__sam_\" ->   <| \"ζ\"->  0.000000000000  , \"τ1\"-> 0.000000000000  , \"τS\"-> 0.000000000000  , \"τN\"-> 0.000000000000  , \"τC\"-> 0.000000000000  , \"κ0\"-> 0.000000000000  , \"mm1\"-> 0.000000000000  , \"mm2\"-> 0.000000000000  , \"mm3\"-> 0.000000000000  , \"T\"->  0.438000000000  , \"B\"-> 8.000000000000  , \"θ\"-> 90.000000000000  |>   , \r\"IDS0354_210906_RAW_cal__ref_\" ->   <| \"ζ\"->  0.035878229865  , \"τ1\"-> 0.020618191238  , \"τS\"-> 0.028341492437  , \"τN\"-> 0.001542437572  , \"τC\"-> 0.002465046672  , \"κ0\"-> 0.000000003272  , \"mm1\"-> 0.000000000000  , \"mm2\"-> 0.000000000000  , \"mm3\"-> 0.000000000000  , \"T\"->  0.530000000000  , \"B\"-> 8.000000000000  , \"θ\"-> 90.000000000000  |>   , \r\"IDS0354_210906_RAW_cal__sam_\" ->   <| \"ζ\"->  0.000000000000  , \"τ1\"-> 0.000000000000  , \"τS\"-> 0.000000000000  , \"τN\"-> 0.000000000000  , \"τC\"-> 0.000000000000  , \"κ0\"-> 0.000000000000  , \"mm1\"-> 0.000000000000  , \"mm2\"-> 0.000000000000  , \"mm3\"-> 0.000000000000  , \"T\"->  0.530000000000  , \"B\"-> 8.000000000000  , \"θ\"-> 90.000000000000  |>   , \r\"IDS0355_210906_RAW_cal__ref_\" ->   <| \"ζ\"->  0.022259133140  , \"τ1\"-> 0.021062021806  , \"τS\"-> 0.021361272182  , \"τN\"-> 0.000526217477  , \"τC\"-> 0.003770290408  , \"κ0\"-> 0.000000005411  , \"mm1\"-> 0.000000000000  , \"mm2\"-> 0.000000000000  , \"mm3\"-> 0.000000000000  , \"T\"->  0.830000000000  , \"B\"-> 8.000000000000  , \"θ\"-> 90.000000000000  |>   , \r\"IDS0355_210906_RAW_cal__sam_\" ->   <| \"ζ\"->  0.000000000000  , \"τ1\"-> 0.000000000000  , \"τS\"-> 0.000000000000  , \"τN\"-> 0.000000000000  , \"τC\"-> 0.000000000000  , \"κ0\"-> 0.000000000000  , \"mm1\"-> 0.000000000000  , \"mm2\"-> 0.000000000000  , \"mm3\"-> 0.000000000000  , \"T\"->  0.830000000000  , \"B\"-> 8.000000000000  , \"θ\"-> 90.000000000000  |>   , \r\"IDS0359_210907_RAW_cal__ref_\" ->   <| \"ζ\"->  0.381003010305  , \"τ1\"-> 0.083336505244  , \"τS\"-> 0.050211621127  , \"τN\"-> 0.550745531665  , \"τC\"-> 0.000692694606  , \"κ0\"-> 0.000000000382  , \"mm1\"-> 0.000000000000  , \"mm2\"-> 0.000000000000  , \"mm3\"-> 0.000000000000  , \"T\"->  0.120000000000  , \"B\"-> 12.000000000000  , \"θ\"-> 60.000000000000  |>   , \r\"IDS0359_210907_RAW_cal__sam_\" ->   <| \"ζ\"->  0.000000000000  , \"τ1\"-> 0.000000000000  , \"τS\"-> 0.000000000000  , \"τN\"-> 0.000000000000  , \"τC\"-> 0.000000000000  , \"κ0\"-> 0.000000000000  , \"mm1\"-> 0.000000000000  , \"mm2\"-> 0.000000000000  , \"mm3\"-> 0.000000000000  , \"T\"->  0.120000000000  , \"B\"-> 12.000000000000  , \"θ\"-> 60.000000000000  |>   , \r\"IDS0360_210907_RAW_cal__ref_\" ->   <| \"ζ\"->  0.323840637004  , \"τ1\"-> 0.072581646931  , \"τS\"-> 0.047951414335  , \"τN\"-> 0.283785405218  , \"τC\"-> 0.000913184933  , \"κ0\"-> 0.000000000636  , \"mm1\"-> 0.000000000000  , \"mm2\"-> 0.000000000000  , \"mm3\"-> 0.000000000000  , \"T\"->  0.150000000000  , \"B\"-> 12.000000000000  , \"θ\"-> 60.000000000000  |>   , \r\"IDS0360_210907_RAW_cal__sam_\" ->   <| \"ζ\"->  0.000000000000  , \"τ1\"-> 0.000000000000  , \"τS\"-> 0.000000000000  , \"τN\"-> 0.000000000000  , \"τC\"-> 0.000000000000  , \"κ0\"-> 0.000000000000  , \"mm1\"-> 0.000000000000  , \"mm2\"-> 0.000000000000  , \"mm3\"-> 0.000000000000  , \"T\"->  0.150000000000  , \"B\"-> 12.000000000000  , \"θ\"-> 60.000000000000  |>   , \r\"IDS0361_210908_RAW_cal__ref_\" ->   <| \"ζ\"->  0.279940228007  , \"τ1\"-> 0.067057240536  , \"τS\"-> 0.048025817643  , \"τN\"-> 0.170011495172  , \"τC\"-> 0.001015047914  , \"κ0\"-> 0.000000000754  , \"mm1\"-> 0.000000000000  , \"mm2\"-> 0.000000000000  , \"mm3\"-> 0.000000000000  , \"T\"->  0.168000000000  , \"B\"-> 12.000000000000  , \"θ\"-> 60.000000000000  |>   , \r\"IDS0361_210908_RAW_cal__sam_\" ->   <| \"ζ\"->  0.000000000000  , \"τ1\"-> 0.000000000000  , \"τS\"-> 0.000000000000  , \"τN\"-> 0.000000000000  , \"τC\"-> 0.000000000000  , \"κ0\"-> 0.000000000000  , \"mm1\"-> 0.000000000000  , \"mm2\"-> 0.000000000000  , \"mm3\"-> 0.000000000000  , \"T\"->  0.168000000000  , \"B\"-> 12.000000000000  , \"θ\"-> 60.000000000000  |>   , \r\"IDS0362_210908_RAW_cal__ref_\" ->   <| \"ζ\"->  0.206594976212  , \"τ1\"-> 0.057885925979  , \"τS\"-> 0.038698575169  , \"τN\"-> 0.092347634602  , \"τC\"-> 0.001108131545  , \"κ0\"-> 0.000000001046  , \"mm1\"-> 0.000000000000  , \"mm2\"-> 0.000000000000  , \"mm3\"-> 0.000000000000  , \"T\"->  0.197000000000  , \"B\"-> 12.000000000000  , \"θ\"-> 60.000000000000  |>   , \r\"IDS0362_210908_RAW_cal__sam_\" ->   <| \"ζ\"->  0.000000000000  , \"τ1\"-> 0.000000000000  , \"τS\"-> 0.000000000000  , \"τN\"-> 0.000000000000  , \"τC\"-> 0.000000000000  , \"κ0\"-> 0.000000000000  , \"mm1\"-> 0.000000000000  , \"mm2\"-> 0.000000000000  , \"mm3\"-> 0.000000000000  , \"T\"->  0.197000000000  , \"B\"-> 12.000000000000  , \"θ\"-> 60.000000000000  |>   , \r\"IDS0363_210908_RAW_cal__ref_\" ->   <| \"ζ\"->  0.123216898961  , \"τ1\"-> 0.041424716624  , \"τS\"-> 0.030606562009  , \"τN\"-> 0.033679175657  , \"τC\"-> 0.001245281919  , \"κ0\"-> 0.000000001353  , \"mm1\"-> 0.000000000000  , \"mm2\"-> 0.000000000000  , \"mm3\"-> 0.000000000000  , \"T\"->  0.250000000000  , \"B\"-> 12.000000000000  , \"θ\"-> 60.000000000000  |>   , \r\"IDS0363_210908_RAW_cal__sam_\" ->   <| \"ζ\"->  0.000000000000  , \"τ1\"-> 0.000000000000  , \"τS\"-> 0.000000000000  , \"τN\"-> 0.000000000000  , \"τC\"-> 0.000000000000  , \"κ0\"-> 0.000000000000  , \"mm1\"-> 0.000000000000  , \"mm2\"-> 0.000000000000  , \"mm3\"-> 0.000000000000  , \"T\"->  0.250000000000  , \"B\"-> 12.000000000000  , \"θ\"-> 60.000000000000  |>   , \r\"IDS0364_210908_RAW_cal__ref_\" ->   <| \"ζ\"->  0.083979493288  , \"τ1\"-> 0.035863468022  , \"τS\"-> 0.027413945050  , \"τN\"-> 0.017174500536  , \"τC\"-> 0.001551957186  , \"κ0\"-> 0.000000001738  , \"mm1\"-> 0.000000000000  , \"mm2\"-> 0.000000000000  , \"mm3\"-> 0.000000000000  , \"T\"->  0.307000000000  , \"B\"-> 12.000000000000  , \"θ\"-> 60.000000000000  |>   , \r\"IDS0364_210908_RAW_cal__sam_\" ->   <| \"ζ\"->  0.000000000000  , \"τ1\"-> 0.000000000000  , \"τS\"-> 0.000000000000  , \"τN\"-> 0.000000000000  , \"τC\"-> 0.000000000000  , \"κ0\"-> 0.000000000000  , \"mm1\"-> 0.000000000000  , \"mm2\"-> 0.000000000000  , \"mm3\"-> 0.000000000000  , \"T\"->  0.307000000000  , \"B\"-> 12.000000000000  , \"θ\"-> 60.000000000000  |>   , \r\"IDS0365_210908_RAW_cal__ref_\" ->   <| \"ζ\"->  0.061526991224  , \"τ1\"-> 0.029624261727  , \"τS\"-> 0.025208021627  , \"τN\"-> 0.009698502183  , \"τC\"-> 0.001918212332  , \"κ0\"-> 0.000000002116  , \"mm1\"-> 0.000000000000  , \"mm2\"-> 0.000000000000  , \"mm3\"-> 0.000000000000  , \"T\"->  0.360000000000  , \"B\"-> 12.000000000000  , \"θ\"-> 60.000000000000  |>   , \r\"IDS0365_210908_RAW_cal__sam_\" ->   <| \"ζ\"->  0.000000000000  , \"τ1\"-> 0.000000000000  , \"τS\"-> 0.000000000000  , \"τN\"-> 0.000000000000  , \"τC\"-> 0.000000000000  , \"κ0\"-> 0.000000000000  , \"mm1\"-> 0.000000000000  , \"mm2\"-> 0.000000000000  , \"mm3\"-> 0.000000000000  , \"T\"->  0.360000000000  , \"B\"-> 12.000000000000  , \"θ\"-> 60.000000000000  |>   , \r\"IDS0366_210908_RAW_cal__ref_\" ->   <| \"ζ\"->  0.045515267447  , \"τ1\"-> 0.026001810196  , \"τS\"-> 0.023136668780  , \"τN\"-> 0.005224117981  , \"τC\"-> 0.002327400857  , \"κ0\"-> 0.000000002646  , \"mm1\"-> 0.000000000000  , \"mm2\"-> 0.000000000000  , \"mm3\"-> 0.000000000000  , \"T\"->  0.430000000000  , \"B\"-> 12.000000000000  , \"θ\"-> 60.000000000000  |>   , \r\"IDS0366_210908_RAW_cal__sam_\" ->   <| \"ζ\"->  0.000000000000  , \"τ1\"-> 0.000000000000  , \"τS\"-> 0.000000000000  , \"τN\"-> 0.000000000000  , \"τC\"-> 0.000000000000  , \"κ0\"-> 0.000000000000  , \"mm1\"-> 0.000000000000  , \"mm2\"-> 0.000000000000  , \"mm3\"-> 0.000000000000  , \"T\"->  0.430000000000  , \"B\"-> 12.000000000000  , \"θ\"-> 60.000000000000  |>   , \r\"IDS0367_210908_RAW_cal__ref_\" ->   <| \"ζ\"->  0.037324451442  , \"τ1\"-> 0.019605264024  , \"τS\"-> 0.021700560504  , \"τN\"-> 0.002800944156  , \"τC\"-> 0.002526998509  , \"κ0\"-> 0.000000003301  , \"mm1\"-> 0.000000000000  , \"mm2\"-> 0.000000000000  , \"mm3\"-> 0.000000000000  , \"T\"->  0.530000000000  , \"B\"-> 12.000000000000  , \"θ\"-> 60.000000000000  |>   , \r\"IDS0367_210908_RAW_cal__sam_\" ->   <| \"ζ\"->  0.000000000000  , \"τ1\"-> 0.000000000000  , \"τS\"-> 0.000000000000  , \"τN\"-> 0.000000000000  , \"τC\"-> 0.000000000000  , \"κ0\"-> 0.000000000000  , \"mm1\"-> 0.000000000000  , \"mm2\"-> 0.000000000000  , \"mm3\"-> 0.000000000000  , \"T\"->  0.530000000000  , \"B\"-> 12.000000000000  , \"θ\"-> 60.000000000000  |>   , \r\"IDS0368_210908_RAW_cal__ref_\" ->   <| \"ζ\"->  0.030581023885  , \"τ1\"-> 0.017326525290  , \"τS\"-> 0.020225378130  , \"τN\"-> 0.001703135365  , \"τC\"-> 0.003380889395  , \"κ0\"-> 0.000000003914  , \"mm1\"-> 0.000000000000  , \"mm2\"-> 0.000000000000  , \"mm3\"-> 0.000000000000  , \"T\"->  0.630000000000  , \"B\"-> 12.000000000000  , \"θ\"-> 60.000000000000  |>   , \r\"IDS0368_210908_RAW_cal__sam_\" ->   <| \"ζ\"->  0.000000000000  , \"τ1\"-> 0.000000000000  , \"τS\"-> 0.000000000000  , \"τN\"-> 0.000000000000  , \"τC\"-> 0.000000000000  , \"κ0\"-> 0.000000000000  , \"mm1\"-> 0.000000000000  , \"mm2\"-> 0.000000000000  , \"mm3\"-> 0.000000000000  , \"T\"->  0.630000000000  , \"B\"-> 12.000000000000  , \"θ\"-> 60.000000000000  |>   , \r\"IDS0369_210908_RAW_cal__ref_\" ->   <| \"ζ\"->  0.022212344829  , \"τ1\"-> 0.017343641344  , \"τS\"-> 0.018001662092  , \"τN\"-> 0.000711569404  , \"τC\"-> 0.004309595418  , \"κ0\"-> 0.000000005439  , \"mm1\"-> 0.000000000000  , \"mm2\"-> 0.000000000000  , \"mm3\"-> 0.000000000000  , \"T\"->  0.830000000000  , \"B\"-> 12.000000000000  , \"θ\"-> 60.000000000000  |>   , \r\"IDS0369_210908_RAW_cal__sam_\" ->   <| \"ζ\"->  0.000000000000  , \"τ1\"-> 0.000000000000  , \"τS\"-> 0.000000000000  , \"τN\"-> 0.000000000000  , \"τC\"-> 0.000000000000  , \"κ0\"-> 0.000000000000  , \"mm1\"-> 0.000000000000  , \"mm2\"-> 0.000000000000  , \"mm3\"-> 0.000000000000  , \"T\"->  0.830000000000  , \"B\"-> 12.000000000000  , \"θ\"-> 60.000000000000  |>   , \r\"IDS0370_210908_RAW_cal__ref_\" ->   <| \"ζ\"->  0.021569402950  , \"τ1\"-> 0.017921737944  , \"τS\"-> 0.015463128015  , \"τN\"-> 0.000390873619  , \"τC\"-> 0.004954240411  , \"κ0\"-> 0.000000007586  , \"mm1\"-> 0.000000000000  , \"mm2\"-> 0.000000000000  , \"mm3\"-> 0.000000000000  , \"T\"->  1.130000000000  , \"B\"-> 12.000000000000  , \"θ\"-> 60.000000000000  |>   , \r\"IDS0370_210908_RAW_cal__sam_\" ->   <| \"ζ\"->  0.000000000000  , \"τ1\"-> 0.000000000000  , \"τS\"-> 0.000000000000  , \"τN\"-> 0.000000000000  , \"τC\"-> 0.000000000000  , \"κ0\"-> 0.000000000000  , \"mm1\"-> 0.000000000000  , 
